vi "fromBooleanSpectrum.vi"(1 "value":bool[](array[boolean]), 2 "attribute name":string, 3 "device name":string) -> (0 "attribute value":T1={"device name"="", "attribute name"="", "quality value"=enum."VALID", "quality string"="", "timestamp"=0.0, "dim. x"=0, "dim. y"=0, "value"=[], "error code"=0, "error stack"=[], "data type"=enum."STRING_SPE"})   [LabVIEW 2014, in "tango.lvlib"]
uses:
  tango.lvlib
  Common VIs/Typedefs/_AttributeValue_t.ctl
  Common VIs/Typedefs/_AttributeQuality_t.ctl
  Common VIs/Typedefs/_AttributeDataType_t.ctl
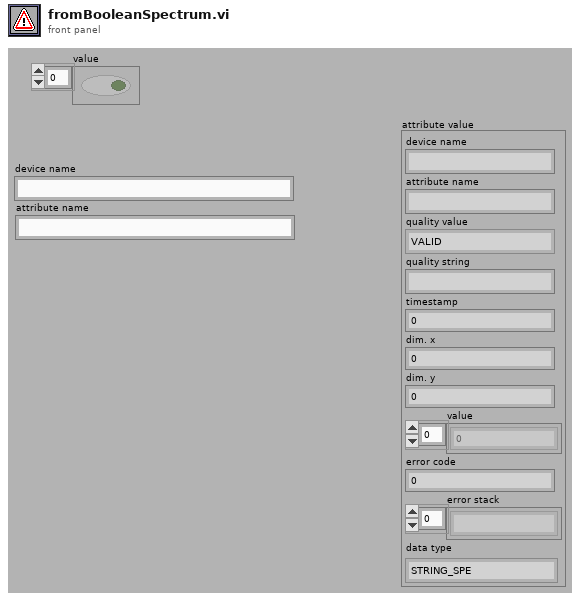
[diagram p1: front panel]
types:
  T1 = typedef "tango.lvlib/_AttributeValue_t.ctl" = cluster{"device name":string, "attribute name":string, "quality value":T2, "quality string":string, "timestamp":dbl, "dim. x":i32, "dim. y":i32, "value":u8[], "error code":i32, "error stack":string[], "data type":T3}
  T2 = typedef "tango.lvlib/_AttributeQuality_t.ctl" = enum16{"VALID", "INVALID", "ALARM", "CHANGING", "UNKNOWN_QUALITY"}
  T3 = typedef "tango.lvlib/_AttributeDataType_t.ctl" = enum16{"STATE_SCA", "STATE_SPE", "STATE_IMG", "STRING_SCA", "STRING_SPE", "STRING_IMG", "BOOL_SCA", "BOOL_SPE", "BOOL_IMG", "UCHAR_SCA", "UCHAR_SPE", "UCHAR_IMG", "SHORT_SCA", "SHORT_SPE", "SHORT_IMG", "USHORT_SCA", "USHORT_SPE", "USHORT_IMG", "LONG_SCA", "LONG_SPE", "LONG_IMG", "ULONG_SCA", "ULONG_SPE", "ULONG_IMG", "LONG64_SCA", "LONG64_SPE", "LONG64_IMG", "ULONG64_SCA", "ULONG64_SPE", "ULONG64_IMG", "FLOAT_SCA", "FLOAT_SPE", "FLOAT_IMG", "DOUBLE_SCA", "DOUBLE_SPE", "DOUBLE_IMG", "UNKNOWN_DATA_TYPE"}
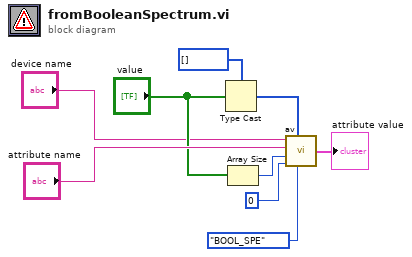
[diagram p0: block diagram]
diagram:
  n1 = Type Cast(type=u8[] [], x="value") -> (*(type *) &x=w7:u8[])
  n2 = Array Size(array="value") -> (size(s)=w6:i32)
  n3 = call "av.vi"("tango data type"=_AttributeDataType_t."BOOL_SPE", "data"=w7, "dim. y"=0, "dim. x"=w6, "attribute name"="attribute name", "device name"="device name") -> ("attribute value"=→"attribute value":T1)
